vi "Get Coordinates.vi"(8 "error in (no error)":errorcluster, 9 "Plot ID":i32, 11 "3D Plot.lvclass in":refnum<class "3D Plot.lvclass">) -> (0 "error out":errorcluster, 1 "Coordinates System":enum16{"Cartesian", "Cylindrical", "Spherical"}(ring), 3 "3D Plot.lvclass out":refnum<class "3D Plot.lvclass">)   [LabVIEW 2020, in "3D Plot.lvclass"]
uses:
  3D Plot.lvclass
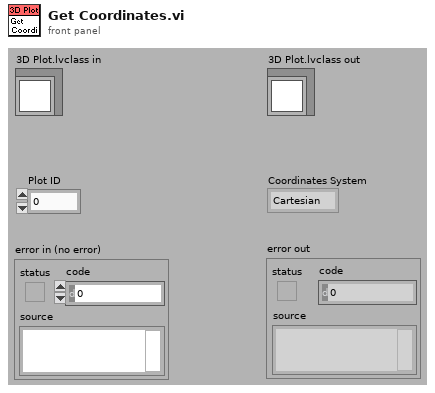
[diagram p1: front panel]
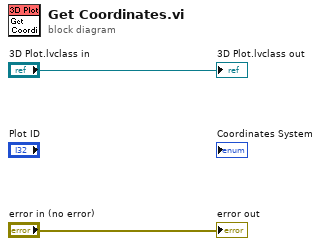
[diagram p0: block diagram]
diagram:
  "3D Plot.lvclass out" <- "3D Plot.lvclass in"
  "error out" <- "error in (no error)"
